vi "Create Array Subset.vi"   [LabVIEW 2012, in "Scripting Tools.lvlib"]
uses:
  Scripting Tools.lvlib
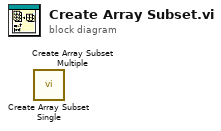
[diagram p0: block diagram]
diagram:
  n1 = call "Create Array Subset Single.vi"() -> ()  [unwired: 9 in, 3 out]
  n2 = call "Create Array Subset Multiple.vi"() -> ()  [unwired: 9 in, 3 out]
